vi "Get_DI.vi"(0 "reference in":refnum<class "DI.lvclass">) -> (6 "DI":bool)   [LabVIEW 2019, in "DI.lvclass"]
uses:
  DI.lvclass
  DI.lvclass/DI.ctl
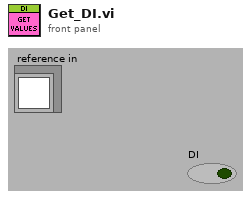
[diagram p1: front panel]
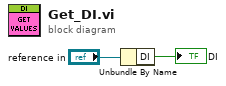
[diagram p0: block diagram]
diagram:
  n1 = Unbundle By Name("reference in") -> ("DI"=→"DI":bool)
